vi "Pa_Mo_Sy_Final.vi"() -> ()   [LabVIEW 2013]
uses:
  <vilib>/Platform/TimedLoop/XDataNode/timing_clust.ctl
  <vilib>/Platform/TimedLoop/XDataNode/nitl_modes.ctl
  <vilib>/Platform/TimedLoop/XDataNode/wakeup.ctl
  <vilib>/userdefined/High Color/IMAQdx.ctl
  <vilib>/MakerHub/LINX/Public/Peripherals/Analog/Analog Read 1 Chan.vi
  <vilib>/MakerHub/LINX/Public/Peripherals/Digital/Digital Read 1 Chan.vi
  <vilib>/MakerHub/LINX/Private/Local IO/LinxI2cWrite.vi
  <vilib>/MakerHub/LINX/Public/Utilities/Check Channel.vi
  <vilib>/MakerHub/LINX/Public/Peripherals/Analog/Analog Read N Chans.vi
  <vilib>/MakerHub/LINX/Public/Peripherals/Digital/Digital Read N Chans.vi
  <vilib>/MakerHub/LINX/Private/Local IO/LinxAnalogRead.vi
  <vilib>/MakerHub/LINX/Private/Local IO/LinxDigitalRead.vi
  <vilib>/MakerHub/LINX/Public/Utilities/Open Serial.vi
  <vilib>/MakerHub/LINX/Private/Utilties/Generate Error.vi
  <vilib>/platform/TimedLoop/XDataNode/XDataNode.xnode
  <vilib>/vision/driver/NI_Vision_Acquisition_Software.lvlib
  <vilib>/MakerHub/LINX/LMH-LINX.lvlib
  <vilib>/Platform/TimedLoop/XDataNode/XDNodeRunTimeDep.lvlib
  <vilib>/Analysis/NI_AALPro.lvlib
panel:
  in  "?":bool
  out "pulse":bool
  out "Report":string
  in  "Activity Factor":string(combo)
  out "Carbohydrates":dbl
  out "Fat":dbl format="%#_3g"
  out "Protein":dbl format="%#_2g"
  out "Calories":dbl format="%#_2g"
  out "BMR":dbl format="%#_2g"
  out "Body Fat":dbl format="%#_2g"
  in  "Blood Sugar":i64
  in  "GSR":bool
  out "Voltage":dbl
  out "Threshold":dbl
  out "Emotion Change":bool
  in  "Temperature":bool
  in  "stop":bool
  out "Date":string
  in  "Patient ID":i64
  in  "Blood Group":string(combo)
  in  "E-Mail":string
  in  "Mobile":i64
  in  "Prescription":string
  in  "Queries/Problems":string
  in  "Diastole":i64
  in  "Systole":i64
  out "BMI":i64
  in  "Weight(kg)":i64 caption="Weight"
  in  "Height(cm)":i64 caption="Height"
  out "Heart Beat":i64
  out "Thermometer(F)":dbl(slide) scale=0.0..110.0
  out "Galvanic Skin Response(GSR)":dbl(graph)
  in  "Sex":string(combo)
  in  "ECG":bool
  out "Electrocardiogram(ECG)":dbl(graph)
  out "Webcam":T1(plugin-control)
  in  "Webcam":bool
  out "Age":i64
  in  "Date Of Birth":timestamp
  in  "Patient Name":string
  # "Blood Pressure"
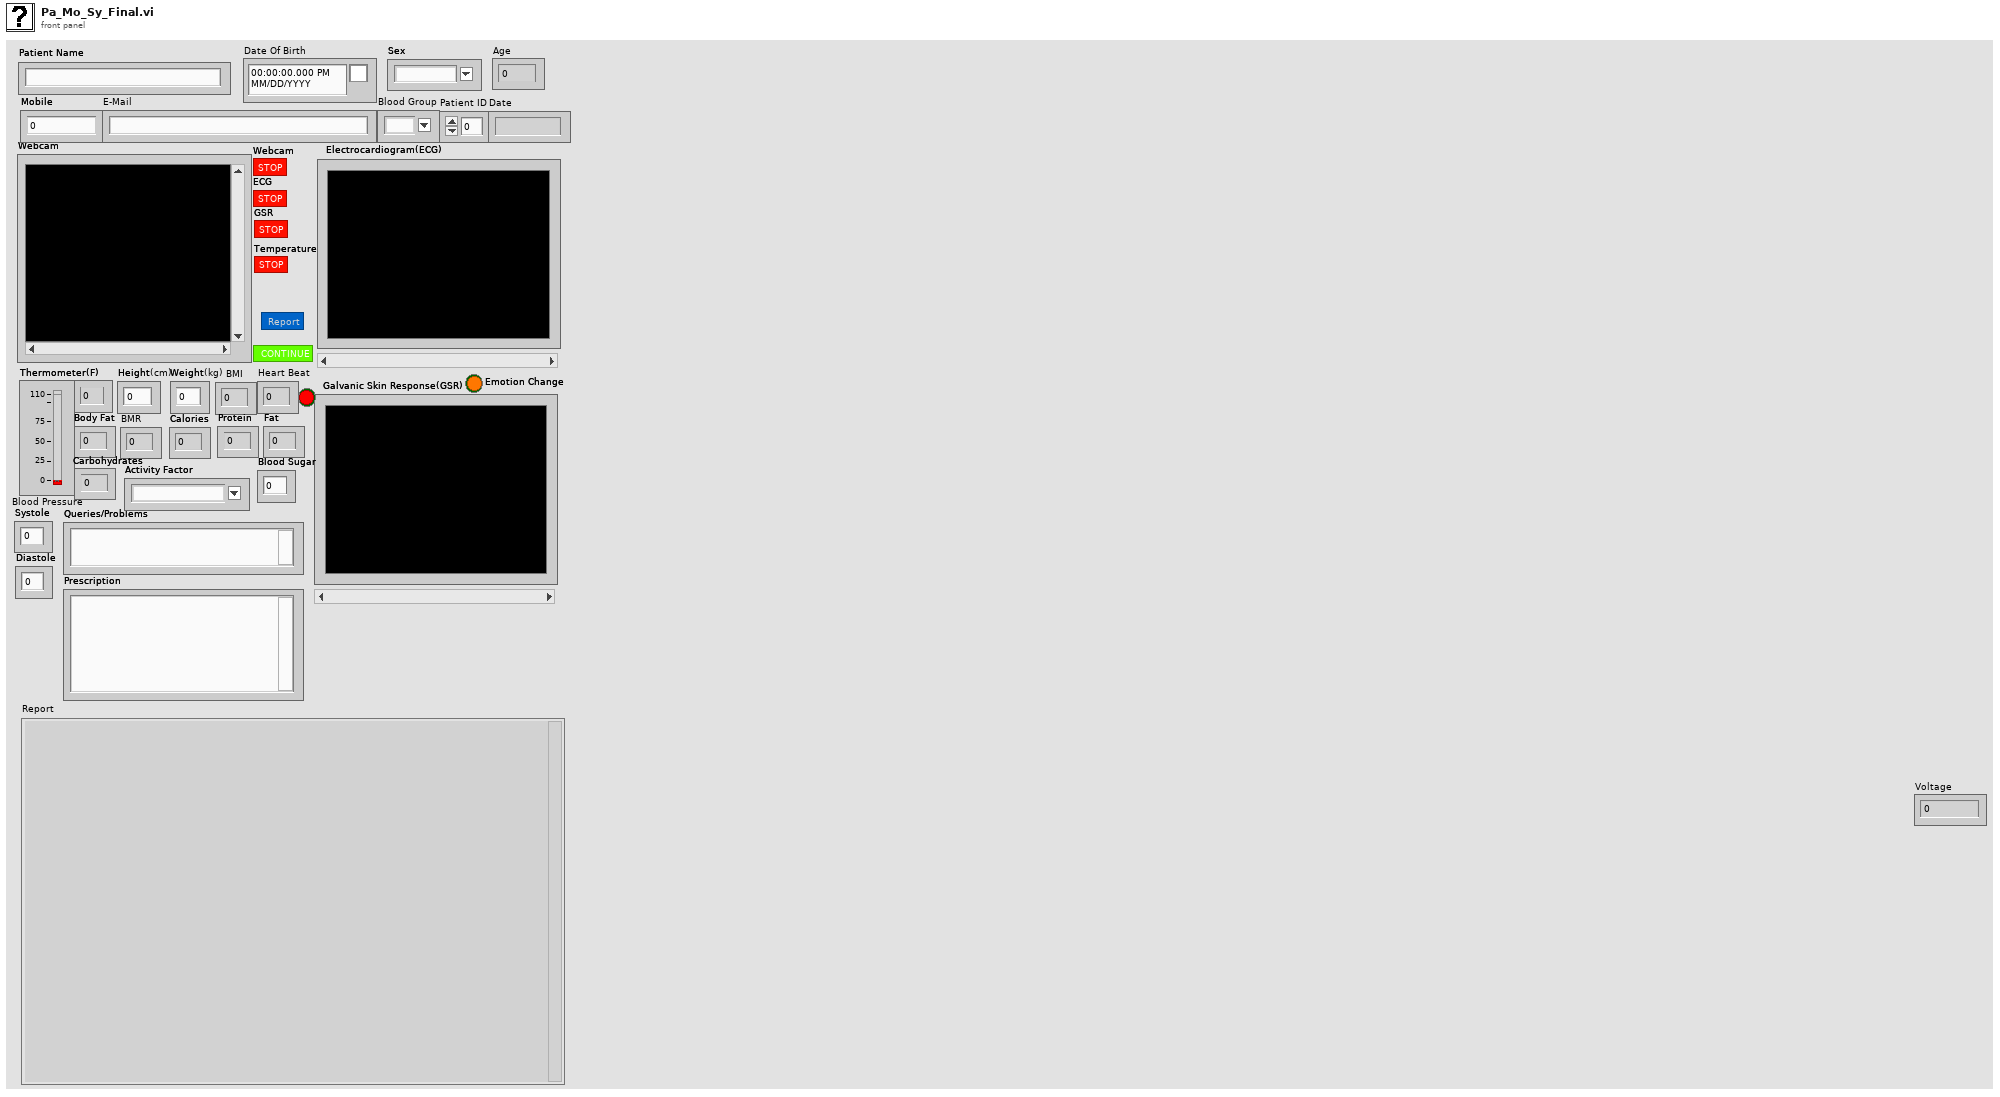
[diagram p1: front panel]
types:
  T1 = typedef "IMAQ Image.ctl" = refnum<image>
  T2 = typedef "XDNodeRunTimeDep.lvlib/timing_clust.ctl" = cluster{"Expected End [f-1]":u64, "Actual End [f-1]":u64, "Finished Late? [f-1]":bool, "Expected End [i-1]":u64, "Actual End [i-1]":u64, "Finished Late? [i-1]":bool, "Expected Start [i]":u64, "Actual Start [i]":u64, "Expected Start [f]":u64, "Actual Start [f]":u64, "Source Name":string, "Structure Name":string, "Period":i64, "Deadline":i64, "Offset":i64, "Start":i64, "Priority":i32, "Timeout":i32, "Mode":T3, "Wakeup Reason":T4, "Error":errorcluster, "Source Type":string, "Secondary Source Type":string, "Global End Time":u64, "Global Start Time":u64, "Frame Duration":u64, "Iteration Duration":u64, "Assigned CPU":i32, "I/O Scan Engine Mode":u32}
  T3 = typedef "XDNodeRunTimeDep.lvlib/nitl_modes.ctl" = enum32{"No Change", "Process missed periods, maintain original phase", "Discard missed periods, maintain original phase", "Process missed periods, ignore original phase", "Discard missed periods, ignore original phase"}
  T4 = typedef "XDNodeRunTimeDep.lvlib/wakeup.ctl" = enum32{"Normal", "Aborted", "Asynchronous wakeup", "Timing source error", "Timed loop error", "Timeout"}
  T5 = typedef "IMAQdx.ctl" = refnum<k21>
  T6 = typedef "LMH-LINX.lvlib/LINX Ref.ctl" = cluster{"IO":T7, "Interface":T8, "LINX Device Config":T9}
  T7 = typedef "LMH-LINX.lvlib/Platform.ctl" = enum16{"Remote", "Local"}
  T8 = typedef "LMH-LINX.lvlib/Interface.ctl" = enum16{"Serial", "TCP"}
  T9 = typedef "LMH-LINX.lvlib/Device.lvlib/LINX Device Config.ctl" = cluster{"Interface":T8, "COM Port":refnum<visa-resource-name>, "TCP Configuration":T10, "Device Family":u8, "Device ID":u8, "Device Name":string, "TCP Ref":refnum<k5>, "Channels":T11}
  T10 = typedef "LMH-LINX.lvlib/Device.lvlib/TCP Config.ctl" = cluster{"IP Address":string, "Port":u16}
  T11 = typedef "LMH-LINX.lvlib/Channels.ctl" = cluster{"DI":u8[], "DO":u8[], "AI":u8[], "AO":u8[], "PWM":u8[], "QE":u8[], "UART":u8[], "I2C 2":u8[], "SPI":u8[], "CAN":u8[], "Servo":u8[], "AI Ref (V)":dbl, "AI Resolution (Bits)":u8, "AO Ref (V)":dbl, "AO Resolution (Bits)":u8}
  T12 = typedef "Image Type" = u32
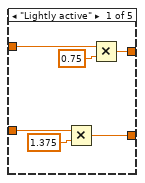
[diagram p3: hidden frame]
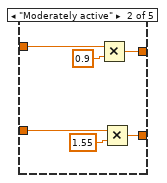
[diagram p4: hidden frame]
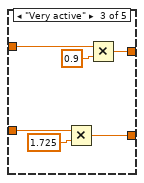
[diagram p5: hidden frame]
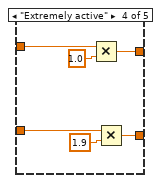
[diagram p6: hidden frame]
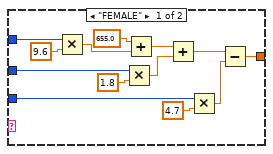
[diagram p7: hidden frame]
diagram:
  n1 = flat-sequence {
    tunnel: [w133] -> w12
    tunnel: [w128] -> w1
    tunnel: w12 -> [w178]
    tunnel: [w178] -> w11
    tunnel: [w177] -> w2
    tunnel: w1 -> [w177]
    tunnel: w11 -> [w182]
    tunnel: [w181] -> w10
    tunnel: [w180] -> w8
    tunnel: w2 -> [w179]
    tunnel: w10 -> [w200]
    tunnel: [w200] -> w9
    tunnel: w8 -> [w199]
    tunnel: [w199] -> w7
    tunnel: w9 -> [w204]
    tunnel: w7 -> [w203]
    tunnel: [w202] -> w6
    tunnel: [w201] -> w4
    tunnel: w6 -> [w250]
    tunnel: [w250] -> w5
    tunnel: w4 -> [w249]
    tunnel: [w249] -> w3
    tunnel: w5 -> [w252]
    tunnel: w3 -> [w251]
    tunnel: [w324] -> w14
    tunnel: [w323] -> w13
    tunnel: w14 -> [_]
    tunnel: w13 -> [w410]
    frame #0 {
      n2 = call "Display Message to User"() -> ("error out"=w15:errorcluster)  [unwired: 10 in, 1 out]
      n3 = invoke on="Queries/Problems" class="Str" method="Reinit To Default"() -> ()  [unwired: 3 in, 3 out]
      n4 = call "Display Message to User2"("error in (no error)"=w15) -> ()  [unwired: 9 in, 2 out]
    }
    frame #1 {
      n5 = while {
        stop <- "?" stop-if-true
      }
    }
    frame #2 {
      n6 = local read "Height(cm)"() -> (w19:i64)
      n7 = local read "Weight(kg)"() -> (w22:i64)
      n8 = Divide(x=w19, y=i64 100) -> (x/y=w18:dbl)
      n9 = Square(x=w18) -> (x^2=w21:dbl)
      n10 = Divide(x=w22, y=w21) -> (x/y=→"BMI":dbl)
    }
    frame #3 {
      w27 = 3 ("offset")
      n11 = Get Date/Time In Seconds() -> (seconds since 1Jan1904=w35:timestamp)
      n12 = Get Date/Time String(seconds (now)=w35) -> (date string=w37:string)  [unwired: 2 in, 1 out]
      "Date" <- w37
      n13 = Get Date/Time String(seconds (now)="Date Of Birth") -> (date string=w36:string)  [unwired: 2 in, 1 out]
      n14 = Decimal String To Number(string=w37, offset=w27) -> (number=w28:i32)  [unwired: 1 in, 1 out]
      n15 = Decimal String To Number(string=w36, offset=w27) -> (number=w29:i32)  [unwired: 1 in, 1 out]
      n16 = Decimal String To Number(string=w37, offset=6) -> (number=w25:i32)  [unwired: 1 in, 1 out]
      n17 = Decimal String To Number(string=w36, offset=6) -> (number=w26:i32)  [unwired: 1 in, 1 out]
      n18 = Less Or Equal?(x=w28, y=w29) -> (x <= y?=w30:bool)
      n19 = Subtract(x=w25, y=w26) -> (x-y=w32:i32)
      n20 = Decrement(x=w32) -> (x-1=w31:i32)
      n21 = Select(t=w31, s=w30, f=w32) -> (s? t:f=→"Age":i32)
    }
    frame #4 {
      n22 = local read "BMI"() -> (w46:i64)
      n23 = local read "Age"() -> (w47:i64)
      n24 = Multiply(x=w46, y=1.2) -> (x*y=w41:dbl)
      n25 = Multiply(x=w47, y=0.23) -> (x*y=w42:dbl)
      n26 = Add(x=w41, y=w42) -> (x+y=w43:dbl)
      n27 = Subtract(x=w43, y=5.4) -> (x-y=w45:dbl)
      n28 = local read "Sex"() -> (w48:string)
      n29 = case shown="\"MALE\", Default" w48 {
        tunnel: w45 -> [w50 w53]
        tunnel: [w50 w51] -> w49
        frame "FEMALE" {
        }
        frame "MALE", Default {
          n30 = Subtract(x=w53, y=10.8) -> (x-y=w51:dbl)
        }
      }
      "Body Fat" <- w49
      n31 = property on="Prescription" class="Str"("Value"="Medicine Name               M/A/E          A/B" ("Prescription")) -> ()  [unwired: 2 in, 2 out]
    }
    frame #5 {
      n32 = local read "Height(cm)"() -> (w69:i64)
      n33 = local read "Weight(kg)"() -> (w61:i64)
      n34 = local read "Age"() -> (w62:i64)
      n35 = local read "Sex"() -> (w60:string)
      n36 = case shown="\"MALE\", Default" w60 {
        tunnel: w61 -> [w103 w125]
        tunnel: w69 -> [w102 w123]
        tunnel: w62 -> [w101 w121]
        tunnel: [w100 w113] -> w64
        frame "FEMALE" {
          n37 = Multiply(x=w103, y=9.6) -> (x*y=w107:dbl)
          n38 = Multiply(x=w102, y=1.8) -> (x*y=w110:dbl)
          n39 = Add(x=655.0, y=w107) -> (x+y=w109:dbl)
          n40 = Add(x=w109, y=w110) -> (x+y=w111:dbl)
          n41 = Multiply(x=w101, y=4.7) -> (x*y=w112:dbl)
          n42 = Subtract(x=w111, y=w112) -> (x-y=w100:dbl)
        }
        frame "MALE", Default {
          n43 = Multiply(x=w125, y=13.7) -> (x*y=w119:dbl)
          n44 = Multiply(x=w123, y=5.0) -> (x*y=w116:dbl)
          n45 = Add(x=66.0, y=w119) -> (x+y=w117:dbl)
          n46 = Add(x=w117, y=w116) -> (x+y=w115:dbl)
          n47 = Multiply(x=w121, y=6.8) -> (x*y=w114:dbl)
          n48 = Subtract(x=w115, y=w114) -> (x-y=w113:dbl)
        }
      }
      "BMR" <- w64
      n49 = Multiply(x=w61, y=2.20462) -> (x*y=w55:dbl)
      n50 = case shown="\"Sedentary\", Default" "Activity Factor" {
        tunnel: w64 -> [w74 w80 w86 w92 w99]
        tunnel: [w73 w79 w85 w91 w97] -> w68
        tunnel: w55 -> [w71 w77 w83 w90 w95]
        tunnel: [w70 w76 w82 w89 w94] -> w56
        frame "Lightly active" {
          n51 = Multiply(x=w74, y=1.375) -> (x*y=w73:dbl)
          n52 = Multiply(x=w71, y=0.75) -> (x*y=w70:dbl)
        }
        frame "Moderately active" {
          n53 = Multiply(x=w77, y=0.9) -> (x*y=w76:dbl)
          n54 = Multiply(x=w80, y=1.55) -> (x*y=w79:dbl)
        }
        frame "Very active" {
          n55 = Multiply(x=w86, y=1.725) -> (x*y=w85:dbl)
          n56 = Multiply(x=w83, y=0.9) -> (x*y=w82:dbl)
        }
        frame "Extremely active" {
          n57 = Multiply(x=w90, y=1.0) -> (x*y=w89:dbl)
          n58 = Multiply(x=w92, y=1.9) -> (x*y=w91:dbl)
        }
        frame "Sedentary", Default {
          n59 = Multiply(x=w95, y=0.4) -> (x*y=w94:dbl)
          n60 = Multiply(x=w99, y=1.2) -> (x*y=w97:dbl)
        }
      }
      "Calories" <- w68
      n61 = Multiply(x=w56, y=4.0) -> (x*y=w67:dbl)
      "Protein" <- w67
      n62 = Multiply(x=w68, y=0.25) -> (x*y=w66:dbl)
      "Fat" <- w66
      n63 = Add(x=w67, y=w66) -> (x+y=w59:dbl)
      n64 = Subtract(x=w68, y=w59) -> (x-y=→"Carbohydrates":dbl)
    }
    frame #6 {
      n65 = call "Display Message to User3"() -> ("error out"=w127:errorcluster)  [unwired: 10 in, 1 out]
      n66 = call "Display Message to User4"("error in (no error)"=w127) -> ("error out"=w126:errorcluster)  [unwired: 9 in, 1 out]
      n67 = call "Display Message to User5"("error in (no error)"=w126) -> ()  [unwired: 9 in, 2 out]
    }
    frame #7 {
      w139 = u8 72  # I2C Slave Address (0)
      w142 = u8 0  # I2C Channel (0)
      n68 = call-poly <vilib>:"Open.vi"("Baud Rate Override"=u32 9600, "Serial Port"=refnum<visa-resource-name> "COM2") -> ("Error Out"=w129:errorcluster, "LINX Resource"=w130:T6)  [unwired: 7 in, 1 out]
      n69 = call <vilib>:"I2C Open.vi"("I2C Channel (0)"=w142, "Error In"=w129, "LINX Resource"=w130) -> ("Error Out"=w134:errorcluster, "LINX Resource"=w135:T6)  [unwired: 7 in]
      n70 = for {
        tunnel: w134 -> [w175]
        tunnel: w135 -> [w174]
        tunnel: w139 -> [w173]
        tunnel: u8[][] [[1, 0], [2, 0], [3, 0]] ("Data") -> [w172] mode=indexing
        tunnel: w142 -> [w171]
        tunnel: [w170] -> w137
        tunnel: [w169] -> w138
        n71 = call <vilib>:"I2C Write.vi"("I2C Channel"=w171, "Error In"=w175, "Data"=w172, "I2C Slave Address (0)"=w173, "LINX Resource"=w174) -> ("Error Out"=w169:errorcluster, "LINX Resource"=w170:T6)  [unwired: 5 in]
      }
      n72 = node-c288() -> (w144:T2)  [unwired: 4 in]
      n73 = timed-loop {
        timing: w144 -> [_]
        timing-out: [_] -> w143
        tunnel: w137 -> [w162]
        tunnel: w138 -> [w161]
        tunnel: w139 -> [w158]
        tunnel: w142 -> [w157]
        tunnel: [w155] -> w141
        tunnel: [w154] -> w140
        stop <- w156 stop-if-true
        n74 = node-c288() -> ()  [unwired: 1 in, 1 out]
        n75 = call <vilib>:"I2C Write.vi"("I2C Channel"=w157, "Error In"=w161, "Data"=u8[] [0], "I2C Slave Address (0)"=w158, "LINX Resource"=w162) -> ("Error Out"=w164:errorcluster, "LINX Resource"=w163:T6)  [unwired: 5 in]
        n76 = call <vilib>:"I2C Read.vi"("I2C Channel"=w157, "Error In"=w164, "Bytes To Read"=u8 16, "I2C Slave Address (0)"=w158, "LINX Resource"=w163) -> ("Error Out"=w155:errorcluster, "Data"=w147:u8[], "LINX Resource"=w154:T6)  [unwired: 4 in]
        n77 = Or(x=w155, y="Temperature") -> (x .or. y?=w156:bool)
        n78 = Index Array(array=w147) -> (element=w153:u8)  [unwired: 1 in]
        n79 = Divide(x=9.0, y=5.0) -> (x/y=w152:dbl)
        n80 = Multiply(x=w153, y=w152) -> (x*y=w149:dbl)
        n81 = Add(x=w149, y=32.0) -> (x+y=→"Thermometer(F)":dbl)
        n82 = node-c288() -> ()  [unwired: 1 in, 1 out]
      }
      n83 = node-c288(w143) -> ()  [unwired: 1 out]
      n84 = call <vilib>:"I2C Close.vi"("I2C Channel (0)"=w142, "Error In"=w141, "LINX Resource"=w140) -> ("Error Out"=w128:errorcluster, "LINX Resource"=w133:T6)  [unwired: 7 in]
    }
    frame #8 {
      n85 = call "Display Message to User6"() -> ("error out"=w176:errorcluster)  [unwired: 10 in, 1 out]
      n86 = call "Display Message to User7"("error in (no error)"=w176) -> ()  [unwired: 9 in, 2 out]
    }
    frame #9 {
      n87 = while {
        tunnel: w182 -> [w197]
        tunnel: [w195] -> w181
        tunnel: [w194] -> w180
        tunnel: [w189] -> w186 mode=indexing
        tunnel: w179 -> [w188]
        stop <- w191 stop-if-true
        n88 = call-poly <vilib>:"Analog Read.vi"("Error In"=w188, "Analog Channel"=u8 2, "LINX Resource"=w197) -> ("Error Out"=w194:errorcluster, "Voltage"=w189:dbl, "LINX Resource"=w195:T6)  [unwired: 5 in, 1 out]
        n89 = local write "Electrocardiogram(ECG)"(w189) -> ()
        n90 = Greater Or Equal?(x=w189, y=2.4) -> (x >= y?=→"pulse":bool)
        n91 = call "Elapsed Time"("Time Target (s)"=20.0) -> ("Time has Elapsed"=w191:bool)  [unwired: 11 in, 7 out]
      }
      n92 = call <vilib>:"Threshold Detector.vi"("threshold"=2.4, "X"=w186) -> ("count"=w187:i32)  [unwired: 1 in, 2 out]
      n93 = Multiply(x=w187, y=3.0) -> (x*y=→"Heart Beat":dbl)
    }
    frame #10 {
      n94 = call "Display Message to User8"() -> ("error out"=w198:errorcluster)  [unwired: 10 in, 1 out]
      n95 = call "Display Message to User9"("error in (no error)"=w198) -> ()  [unwired: 9 in, 2 out]
    }
    frame #11 {
      n96 = flat-sequence {
        tunnel: [w212] -> w207
        tunnel: [w211] -> w206
        tunnel: [w210] -> w205
        tunnel: w204 -> [w209]
        tunnel: w203 -> [w208]
        tunnel: w207 -> [w232]
        tunnel: w206 -> [w231]
        tunnel: [w230] -> w202
        tunnel: [w229] -> w201
        tunnel: w205 -> [w228]
        frame #0 {
          n97 = for {
            N: 500 -> [_]
            shift-right: [w227] -> w214
            shift-left: 0.0 -> [w226]
            tunnel: [w222] -> w212
            tunnel: [w221] -> w211
            tunnel: [w220] -> w210
            tunnel: w209 -> [w219]
            tunnel: w208 -> [w218]
            w220 = u8 1 ("Analog Channel")
            n98 = call-poly <vilib>:"Analog Read.vi"("Error In"=w218, "Analog Channel"=w220, "LINX Resource"=w219) -> ("Error Out"=w221:errorcluster, "Voltage"=w223:dbl, "LINX Resource"=w222:T6)  [unwired: 5 in, 1 out]
            n99 = Multiply(x=w223, y=310.3) -> (x*y=w224:dbl)
            n100 = Add(x=w224, y=w226) -> (x+y=w227:dbl)
          }
          n101 = Divide(x=w214, y=500.0) -> (x/y=→"Threshold":dbl)
        }
        frame #1 {
          n102 = while {
            tunnel: w232 -> [w241]
            tunnel: w231 -> [w240]
            tunnel: [w238] -> w230
            tunnel: [w237] -> w229
            tunnel: w228 -> [w236]
            stop <- "GSR" stop-if-true
            n103 = call-poly <vilib>:"Analog Read.vi"("Error In"=w240, "Analog Channel"=w236, "LINX Resource"=w241) -> ("Error Out"=w237:errorcluster, "Voltage"=w239:dbl, "LINX Resource"=w238:T6)  [unwired: 5 in, 1 out]
            "Voltage" <- w239
            n104 = Wait (ms)(milliseconds to wait=u32 500 ("millisecond timer value")) -> ()  [unwired: 1 out]
            n105 = local read "Threshold"() -> (w244:dbl)
            n106 = Multiply(x=w239, y=310.3) -> (x*y=w234:dbl)
            "Galvanic Skin Response(GSR)" <- w234
            n107 = Subtract(x=w234, y=w244) -> (x-y=w247:dbl)
            n108 = Absolute Value(x=w247) -> (abs(x)=w246:dbl)
            n109 = Greater?(x=w246, y=50.0) -> (0:→"Emotion Change":bool)
          }
        }
      }
    }
    frame #12 {
      n110 = call "Display Message to User10"() -> ("error out"=w248:errorcluster)  [unwired: 10 in, 1 out]
      n111 = call "Display Message to User11"("error in (no error)"=w248) -> ()  [unwired: 9 in, 2 out]
    }
    frame #13 {
      n112 = while {
        tunnel: [w259] -> w253
        tunnel: [w258] -> w254
        tunnel: w252 -> [w257]
        tunnel: w251 -> [w256]
        stop <- "ECG" stop-if-true
        n113 = flat-sequence {
          tunnel: [w272] -> w266
          tunnel: [w271] -> w265
          tunnel: [w269] -> w264
          tunnel: w257 -> [w268]
          tunnel: w256 -> [w267]
          tunnel: w266 -> [w279]
          tunnel: [w278] -> w263
          tunnel: w265 -> [w277]
          tunnel: [w276] -> w262
          tunnel: [w274] -> w261
          tunnel: [w273] -> w260
          tunnel: w264 -> [w273]
          tunnel: w263 -> [w286]
          tunnel: [w285] -> w259
          tunnel: [w284] -> w258
          tunnel: w262 -> [w283]
          tunnel: w261 -> [w281]
          tunnel: w260 -> [w280]
          frame #0 {
            n114 = call-poly <vilib>:"Digital Read.vi"("Error In"=w267, "DI Channel"=u8 2, "LINX Resource"=w268) -> ("Error Out"=w271:errorcluster, "DI Value"=w269:bool, "LINX Resource"=w272:T6)  [unwired: 6 in]
          }
          frame #1 {
            n115 = call-poly <vilib>:"Digital Read.vi"("Error In"=w277, "DI Channel"=u8 3, "LINX Resource"=w279) -> ("Error Out"=w276:errorcluster, "DI Value"=w274:bool, "LINX Resource"=w278:T6)  [unwired: 6 in]
          }
          frame #2 {
            n116 = Or(x=w280, y=w281) -> (x .or. y?=w282:bool)
            n117 = case shown="True" w282 {
              tunnel: [w288 w293] -> w285
              tunnel: w286 -> [w288 w294]
              tunnel: [w287 w291] -> w284
              tunnel: w283 -> [w287 w292]
              frame False {
              }
              frame True {
                n118 = call-poly <vilib>:"Analog Read.vi"("Error In"=w292, "Analog Channel"=u8 0, "LINX Resource"=w294) -> ("Error Out"=w291:errorcluster, "Voltage"=→"Electrocardiogram(ECG)":dbl, "LINX Resource"=w293:T6)  [unwired: 5 in, 1 out]
              }
            }
          }
        }
      }
      n119 = call <vilib>:"Close.vi"("Error In"=w254, "LINX Resource"=w253) -> ()  [unwired: 9 in, 1 out]
    }
    frame #14 {
      n120 = call "Display Message to User12"() -> ()  [unwired: 10 in, 2 out]
    }
    frame #15 {
      w300 = T12 4 items=["Grayscale (U8)", "Grayscale (I16)", "Grayscale (SGL)", "Complex (CSG)", "RGB (U32)", "HSL (U32)", "RGB (U64)", "Grayscale (U16)"] ("Image Type")
      n121 = call <vilib>:"IMAQdx Open Camera.vi"("Session In"=T5 "cam0") -> ("error out"=w296:errorcluster, "Session Out"=w298:T5)  [unwired: 9 in]
      n122 = call "IMAQ Create"("Image Name"="untitled", "Image Type"=w300, "error in (no error)"=w296) -> ("New Image"=w303:T1, "error out"=w297:errorcluster)  [unwired: 1 in, 1 out]
      n123 = call <vilib>:"IMAQdx Configure Grab.vi"("error in"=w297, "Session In"=w298) -> ("error out"=w302:errorcluster, "Session Out"=w301:T5)  [unwired: 8 in]
      n124 = flat-sequence {
        tunnel: w301 -> [w312]
        tunnel: w302 -> [w311]
        tunnel: w303 -> [w310]
        tunnel: [w309] -> w307
        tunnel: [w308] -> w306
        tunnel: [w322] -> w304
        tunnel: w307 -> [w322]
        tunnel: w306 -> [w321]
        tunnel: [w320] -> w305
        frame #0 {
          n125 = while {
            tunnel: w312 -> [w319]
            tunnel: [w318] -> w309
            tunnel: w311 -> [w317]
            tunnel: [w316] -> w308
            tunnel: w310 -> [w315]
            stop <- "Webcam" stop-if-true
            n126 = call <vilib>:"IMAQdx Grab.vi"("error in"=w317, "Image In"=w315, "Session In"=w319) -> ("error out"=w316:errorcluster, "Image Out"=→"Webcam":T1, "Session Out"=w318:T5)  [unwired: 5 in, 1 out]
          }
        }
        frame #1 {
          n127 = invoke on="Webcam" class="ImageControl" method="Reinit To Default"(error in=w321) -> (error out=w320:errorcluster)  [unwired: 2 in, 2 out]
        }
      }
      n128 = call <vilib>:"IMAQdx Close Camera.vi"("error in"=w305, "Session In"=w304) -> ()  [unwired: 9 in, 1 out]
    }
    frame #16 {
      n129 = call "Display Message to User13"() -> ()  [unwired: 10 in, 2 out]
    }
    frame #17 {
      w324 = path "D:/final year project/VIs/PATIENT REPORT.txt" ("file (use dialog)")
      n130 = while {
        tunnel: [w354] -> w323
        stop <- "stop" stop-if-true
        w326 = "cal/day" ("input 25")
        w349 = " mm/Hg  " ("input 55")
        w335 = "********************************************************************************" ("initial string")
        w327 = "\r\n"
        n131 = local read "Thermometer(F)"() -> (w370:dbl)
        n132 = local read "Heart Beat"() -> (w385:i64)
        n133 = Number To Fractional String(number=w370, precision (6)=i16 2) -> (F-format string=w356:string)  [unwired: 2 in]
        n134 = local read "Carbohydrates"() -> (w358:dbl)
        n135 = local read "Body Fat"() -> (w366:dbl)
        n136 = local read "Calories"() -> (w364:dbl)
        n137 = local read "Protein"() -> (w362:dbl)
        n138 = local read "BMR"() -> (w368:dbl)
        n139 = local read "Date"() -> (w388:string)
        n140 = local read "Age"() -> (w394:i64)
        n141 = local read "BMI"() -> (w375:i64)
        n142 = local read "Fat"() -> (w360:dbl)
        n143 = Format Into String(initial string=" ********************************************************************************", w327, "DR.Z.Xxxxxxx Yyyyy,MBBS" ("input 1"), w327, "ABC Hospital,Street,City,State-620006" ("input 2"), w327, "Ph:0431-2431329" ("input 3"), "                         ", "E-Mail:xxxxxx123456@zzzz.com", w327, w335, w327, "Patient Name  :" ("input 12"), "Patient Name", w327, "Age           :", w394, "               ", "Sex           :" ("input 17"), "Sex", w327, "Patient Mobile:" ("input 20"), "Mobile", "       ", "E-Mail        :" ("input 23"), "E-Mail", w327, w335, w327, "Patient ID    :" ("input 28"), "Patient ID", "               ", "Date          :" ("input 31"), w388, w327, w335, w327, "Heartbeat Rate:" ("input 37"), w385, " bpm            ", "Blood Group   :" ("input 40"), "Blood Group", w327, "Height        :" ("input 43"), "Height(cm)", "cm             ", "Weight        :" ("input 46"), "Weight(kg)", "cm", w327, "BMI           :" ("input 49"), w375, "%               ", "Temperature   :" ("input 52"), w356) -> (resulting string=w355:string)  [unwired: 2 in, 1 out]
        n144 = Number To Fractional String(number=w360, precision (6)=i16 2) -> (F-format string=w337:string)  [unwired: 2 in]
        n145 = Number To Fractional String(number=w368, precision (6)=i16 2) -> (F-format string=w344:string)  [unwired: 2 in]
        n146 = Number To Fractional String(number=w366, precision (6)=i16 2) -> (F-format string=w333:string)  [unwired: 2 in]
        n147 = Number To Fractional String(number=w364, precision (6)=i16 2) -> (F-format string=w341:string)  [unwired: 2 in]
        n148 = Number To Fractional String(number=w362, precision (6)=i16 2) -> (F-format string=w339:string)  [unwired: 2 in]
        n149 = Number To Fractional String(number=w358, precision (6)=i16 2) -> (F-format string=w328:string)  [unwired: 2 in]
        n150 = Format Into String(initial string=w355, " C" ("input 55"), w327, "Blood Pressure:" ("input 55"), "Systole", w349, "Diastole", w349, w327, "Blood Sugar   :" ("input 55"), "Blood Sugar", "mg/dL          ", "BMR           :" ("input 55"), w344, "cal/day" ("input 14"), w327, "Body Fat      :" ("input 55"), w333, "%" ("input 18"), "           ", "Calories      :" ("input 55"), w341, w327, "Protein :" ("input 55"), w339, w326, "  ", "Fat :" ("input 55"), w337, w326, "  ", "Carbohydrate :" ("input 55"), w328, w326, w327, w335, w327, "Prescription") -> (resulting string=w354:string)  [unwired: 2 in, 1 out]
      }
      n151 = Write to Text File(file (use dialog)=w324, text=w323) -> ()  [unwired: 2 in, 3 out]
    }
    frame #18 {
      "Report" <- w410
    }
    frame #19 {
      n152 = call "Display Message to User14"() -> ()  [unwired: 10 in, 2 out]
    }
  }
